vi "open_db.vi"(8 "error in (no error)":errorcluster, 11 "DB in":refnum<class "Base de Datos.lvclass">) -> (0 "error out":errorcluster, 3 "DB out":refnum<class "Base de Datos.lvclass">)   [LabVIEW 2019, in "Base de Datos.lvclass"]
uses:
  Base de Datos.lvclass
  Base de Datos.lvclass/Base de Datos.ctl
  <vilib>/Utility/config.llb/Read Key (String).vi
  SQLiteConnector/SQLiteConnection.lvclass
  <vilib>/Utility/config.llb/NI_LVConfig.lvlib
panel:
  out "RutaBD":string
  # "Open Data reference"
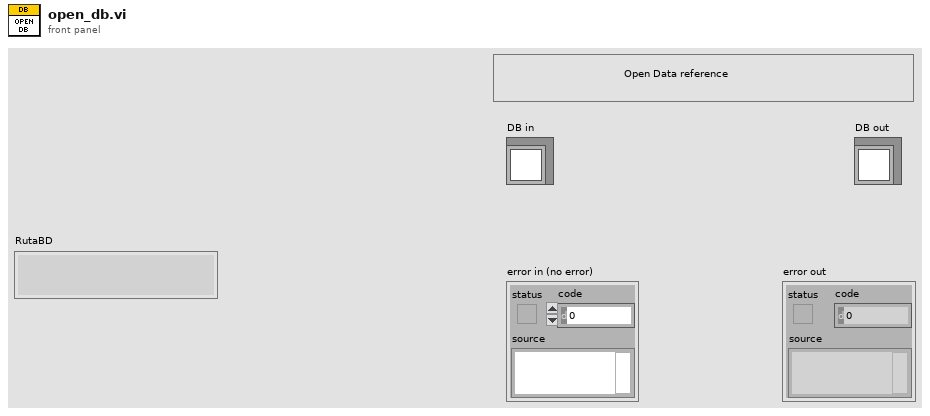
[diagram p1: front panel]
types:
  T1 = typedef "NI_LVConfig.lvlib/Config Data RefNum.ctl" = refnum<k1>
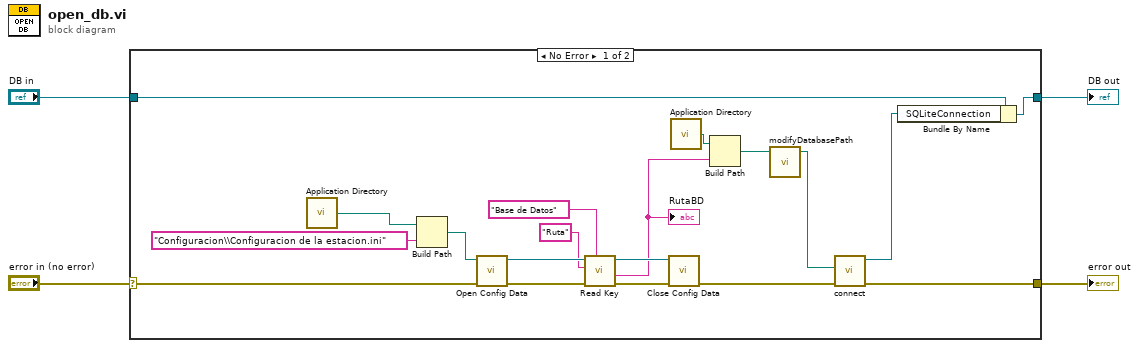
[diagram p0: block diagram]
diagram:
  n1 = case shown="No Error" "error in (no error)" {
    selector: "error in (no error)" -> [w7 w25]
    tunnel: [w23 w25] -> w4
    tunnel: [w21 w24] -> w2
    tunnel: "DB in" -> [w22 w24]
    frame No Error {
      n2 = call <vilib>:"Application Directory.vi"() -> ("Application Directory"=w18:path)
      n3 = Build Path(base path=w18, name or relative path="Configuracion\\Configuracion de la estacion.ini") -> (appended path=w11:path)
      n4 = call <vilib>:"Open Config Data.vi"("error in (no error)"=w7, "configuration file path"=w11) -> ("error out"=w17:errorcluster, "refnum"=w16:T1)  [unwired: 7 in, 1 out]
      n5 = call-poly <vilib>:"Read Key.vi"("section"="Base de Datos", "error in (no error)"=w17, "key"="Ruta", "refnum"=w16) -> ("error out"=w15:errorcluster, "value"=w8:string, "refnum out"=w14:T1)  [unwired: 4 in, 1 out]
      "RutaBD" <- w8
      n6 = call <vilib>:"Close Config Data.vi"("error in (no error)"=w15, "refnum"=w14) -> ("error out"=w6:errorcluster)  [unwired: 8 in, 1 out]
      n7 = call <vilib>:"Application Directory.vi"() -> ("Application Directory"=w10:path)
      n8 = Build Path(base path=w10, name or relative path=w8) -> (appended path=w9:path)
      n9 = call "modifyDatabasePath.vi"("Database Path In"=w9) -> ("Database Path Out"=w5:path)  [unwired: 4 in]
      n10 = call "connect.vi"("error in (no error)"=w6, "Database Path"=w5) -> ("error out"=w23:errorcluster, "object out"=w20:refnum<class "SQLiteConnection.lvclass">)  [unwired: 8 in]
      n11 = Bundle By Name(cluster=w22, "SQLiteConnection"=w20) -> (w21:refnum<class "Base de Datos.lvclass">)
    }
    frame Error {
    }
  }
  "error out" <- w4
  "DB out" <- w2
